vi "Set Shooter Config.vi"(2 "POV Joystick Input":i32) -> ()   [LabVIEW 2020]
uses:
  <vilib>/Rock Robotics/WPI/Solenoid/WPI_SolenoidValue.ctl
  2022 CyberTooth Kokomo/Global Shooter Speed.vi
  <vilib>/Rock Robotics/WPI/Solenoid/WPI_SolenoidSetEnum.vi
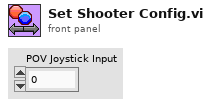
[diagram p1: front panel]
types:
  T1 = typedef "WPI_SolenoidValue.ctl" = enum16{"Off", "On", "Forward", "Reverse"}
  T2 = typedef "WPI_SolenoidDevRef.ctl" = cluster{"DevStatus":errorcluster, "Pneumatics Control Module":u8, "Forward Solenoid Channel":T3, "Reverse Solenoid Channel":T3}
  T3 = typedef "WPI_SolenoidChannel.ctl" = enum8{"Solenoid 0", "Solenoid 1", "Solenoid 2", "Solenoid 3", "Solenoid 4", "Solenoid 5", "Solenoid 6", "Solenoid 7", "Solenoid 8", "Solenoid 9", "Solenoid 10", "Solenoid 11", "Solenoid 12", "Solenoid 13", "Solenoid 14", "Solenoid 15", "Invalid"}
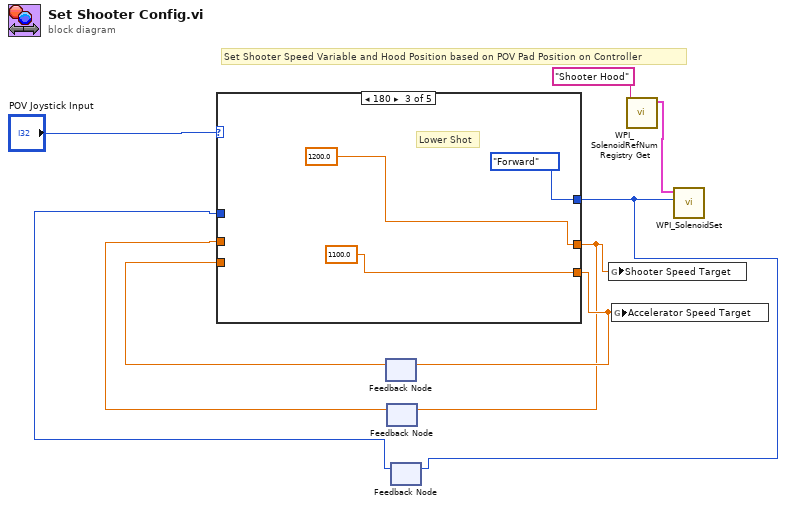
[diagram p0: block diagram]
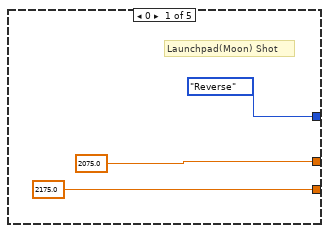
[diagram p2: hidden frame]
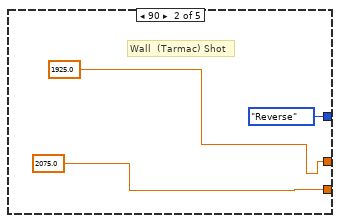
[diagram p3: hidden frame]
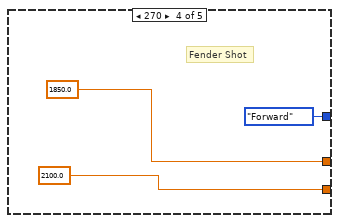
[diagram p4: hidden frame]
diagram:
  # "Set Shooter Speed Variable and Hood Position based on POV Pad Position on Controller"
  n1 = feedback #1() -> (w5:dbl)  [unwired: 1 in]
  n2 = feedback #2() -> (w3:dbl)  [unwired: 1 in]
  n3 = feedback #3() -> (w1:T1)  [unwired: 1 in]
  n4 = case shown="180" "POV Joystick Input" {
    tunnel: [WPI_SolenoidValue."Reverse" ("Value") WPI_SolenoidValue."Reverse" ("Value") WPI_SolenoidValue."Forward" ("Value") WPI_SolenoidValue."Forward" ("Value") w24] -> w2
    tunnel: [2075.0 1925.0 1200.0 1850.0 w23] -> w4
    tunnel: [2175.0 ("Accelerator Speed Target") 2075.0 ("Accelerator Speed Target") 1100.0 ("Accelerator Speed Target") 2100.0 ("Accelerator Speed Target") w22] -> w6
    tunnel: w5 -> [_ _ _ _ w22]
    tunnel: w3 -> [_ _ _ _ w23]
    tunnel: w1 -> [_ _ _ _ w24]
    frame 0 {
      # "Launchpad(Moon) Shot"
    }
    frame 90 {
      # "Wall  (Tarmac) Shot"
    }
    frame 180 {
      # "Lower Shot"
    }
    frame 270 {
      # "Fender Shot"
    }
    frame -1, Default {
    }
  }
  n5 = feedback-in #1(w6) -> ()
  n6 = feedback-in #2(w4) -> ()
  n7 = feedback-in #3(w2) -> ()
  n8 = global write "Global Shooter Speed.vi" "Shooter Speed Target"(w4) -> ()
  n9 = global write "Global Shooter Speed.vi" "Accelerator Speed Target"(w6) -> ()
  n10 = call <vilib>:"WPI_SolenoidRefNum Registry Get.vi"("refnum name"="Shooter Hood") -> ("SolenoidDevRef"=w8:T2)  [unwired: 9 in, 1 out]
  n11 = call-poly <vilib>:"WPI_SolenoidSet.vi"("Value"=w2, "SolenoidDevRef"=w8) -> ()  [unwired: 8 in, 2 out]
